vi "ClearColumnColorOf2DListCtrl.vi"(10 "column":u16, 11 "ArrayRef in":refnum<vi>) -> (3 "ArrayRef out":refnum<vi>)   [LabVIEW 2018, in "Library-Ctrl.lvlib"]
uses:
  Library-Ctrl.lvlib
  <vilib>/Utility/miscctls.llb/LVRowAndColumnTypeDef.ctl
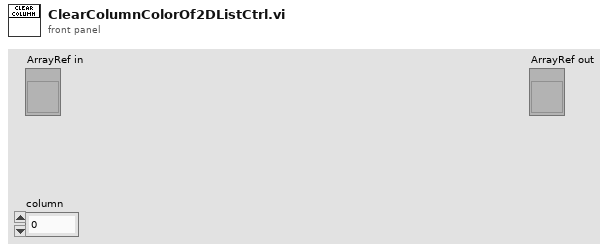
[diagram p1: front panel]
types:
  T1 = typedef "LVRowAndColumnTypeDef.ctl" = cluster{"Row":i32, "Column":i32}
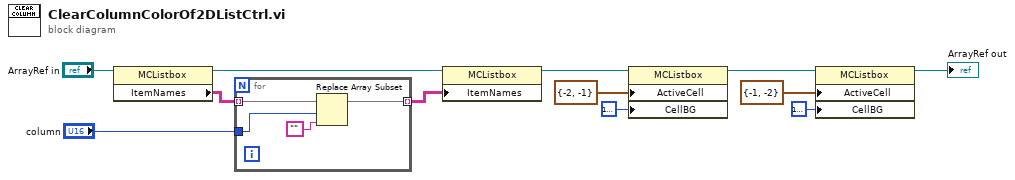
[diagram p0: block diagram]
diagram:
  n1 = property class="MCListbox"(reference="ArrayRef in") -> (reference out=w11:refnum<vi>, "ItemNames"=w12:string[][])  [unwired: 1 in, 1 out]
  n2 = for {
    tunnel: w12 -> [w16] mode=indexing
    tunnel: [w14] -> w10 mode=indexing
    tunnel: "column" -> [w13]
    n3 = Replace Array Subset(array=w16, new element="", index=w13) -> (w14:string[])
  }
  n4 = property class="MCListbox"(reference=w11, "ItemNames"=w10) -> (reference out=w4:refnum<vi>)  [unwired: 1 in, 1 out]
  n5 = property class="MCListbox"(reference=w4, "ActiveCell"=T1 {"Row"=-2, "Column"=-1} ("활성 셀:활성 셀"), "CellBG"=u32 16777222 ("color")) -> (reference out=w3:refnum<vi>)  [unwired: 1 in, 1 out]
  n6 = property class="MCListbox"(reference=w3, "ActiveCell"=T1 {"Row"=-1, "Column"=-2} ("활성 셀:활성 셀"), "CellBG"=u32 16777222 ("color")) -> (reference out=→"ArrayRef out":refnum<vi>)  [unwired: 1 in, 1 out]
